vi "Field Data Manager.vi"(6 "Owning Write":bool, 8 "Increment Sequence":bool, 9 "Operation":T4(ring), 10 "Field Value In":T1, 11 "Field ID":T5) -> (0 "Equal":bool, 2 "Field Value Out":T1)   [LabVIEW 2017]
doc: "Implements the data access operations for the variable table. It supports write, read, assign, and setting flags."
uses:
  <vilib>/Rock Robotics/Network Tables/Field ID.ctl
  <vilib>/Rock Robotics/Network Tables/Field Data.ctl
  <vilib>/Rock Robotics/Network Tables/Field Type.ctl
  <vilib>/Rock Robotics/Network Tables/Sequence.ctl
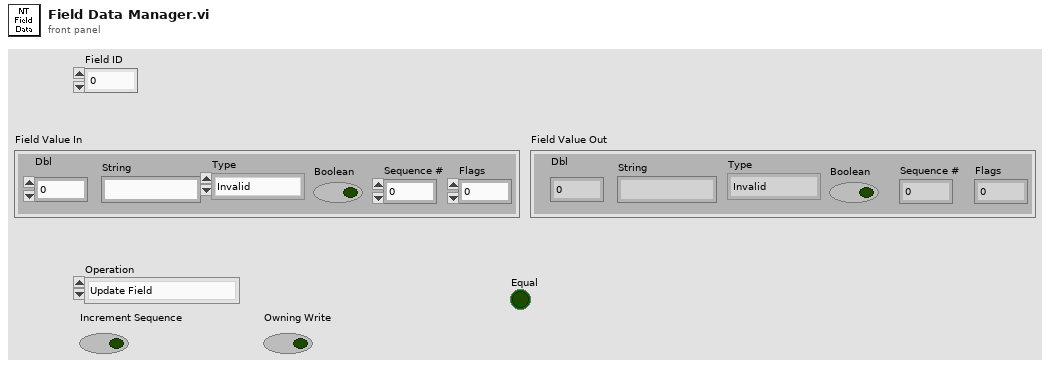
[diagram p1: front panel]
types:
  T1 = typedef "Field Data.ctl" = cluster{"Dbl":dbl, "String":string, "Type":T2, "Boolean":bool, "Sequence #":T3, "Flags":u8}
  T2 = typedef "Field Type.ctl" = enum8{"Invalid", "Bool", "Numeric", "String", "Raw", "Boolean Array", "Numeric Array", "String Array", "RPC"}
  T3 = typedef "Sequence.ctl" = u16
  T4 = enum16{"Update Field", "Read Field", "Assign Field", "Remove All", "Set Persistence", "Clear Persistence"}
  T5 = typedef "Field ID.ctl" = i32
  T6 = cluster{"Dbl":bool, "String":bool, "Type":bool, "Boolean":bool, "Sequence #":bool, "Flags":bool}
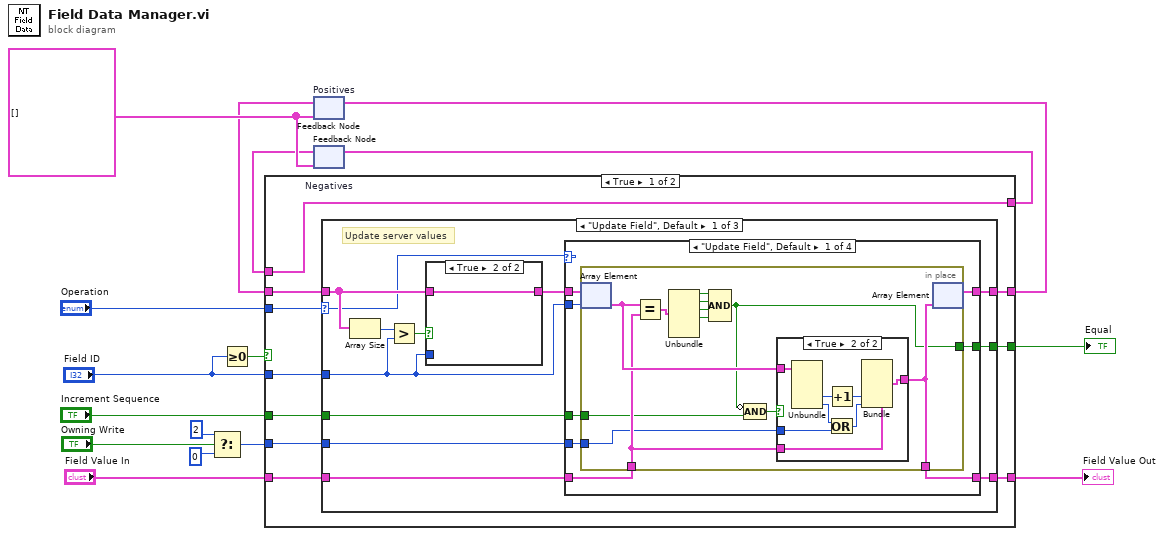
[diagram p0: block diagram]
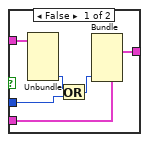
[diagram p2: hidden frame]
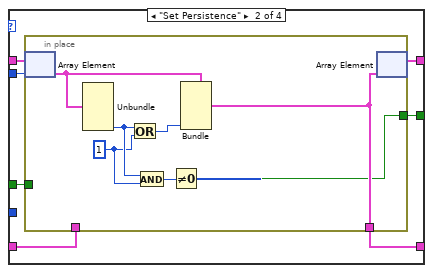
[diagram p3: hidden frame]
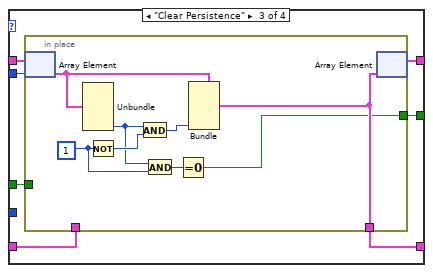
[diagram p4: hidden frame]
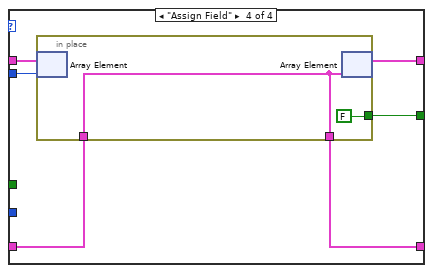
[diagram p5: hidden frame]
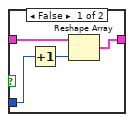
[diagram p6: hidden frame]
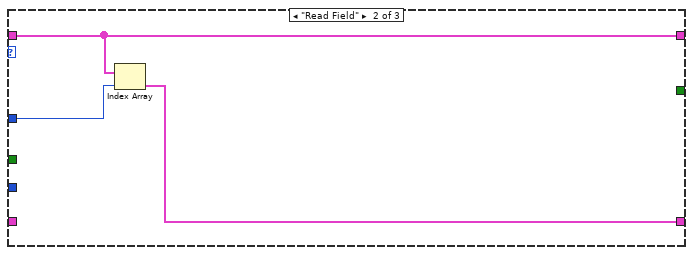
[diagram p7: hidden frame]
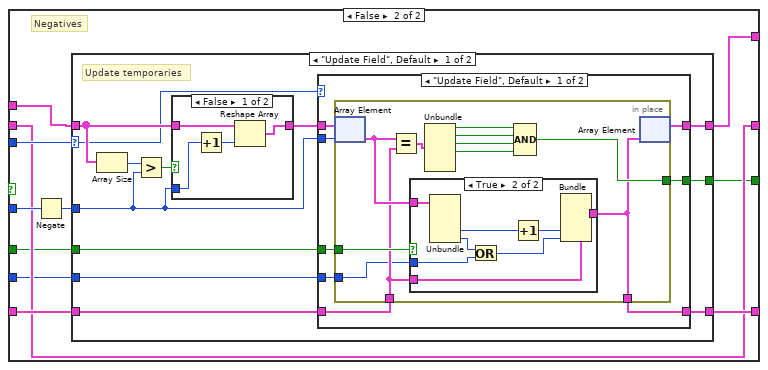
[diagram p9: hidden frame]
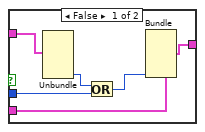
[diagram p10: hidden frame]
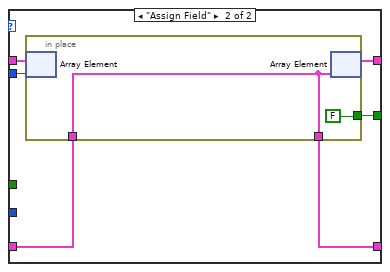
[diagram p11: hidden frame]
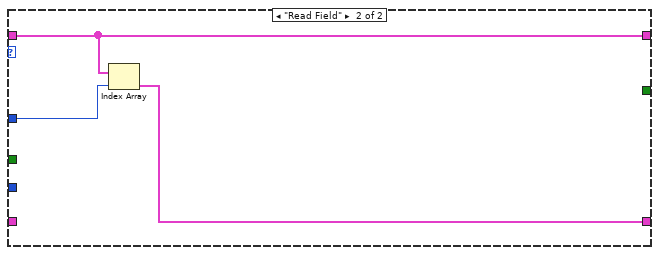
[diagram p13: hidden frame]
diagram:
  w12 = T1[] []
  n1 = Select(t=u8 2, s="Owning Write", f=u8 0) -> (s? t:f=w1:u8)
  n2 = Greater Or Equal To 0?(x="Field ID") -> (x >= 0?=w5:bool)
  n3 = feedback #1 "Positives"(w12) -> (w9:T1[])
  n4 = feedback #2 "Negatives"(w12) -> (w7:T1[])
  n5 = case shown="True" w5 {
    tunnel: "Operation" -> [w26 w129]
    tunnel: "Field Value In" -> [w25 w128]
    tunnel: w9 -> [w24 w123]
    tunnel: [w23 w127] -> w14
    tunnel: [w22 w123] -> w8
    tunnel: "Field ID" -> [w21 w126]
    tunnel: [w20 w124] -> w6
    tunnel: w7 -> [w20 w125]
    tunnel: [w19 w121] -> w11
    tunnel: "Increment Sequence" -> [w18 w120]
    tunnel: w1 -> [w17 w119]
    frame True {
      n6 = case shown="\"Update Field\", Default" w26 {
        selector: w26 -> [w29 _ _]
        tunnel: w25 -> [w36 _ w118]
        tunnel: w24 -> [w34 w115 _]
        tunnel: w21 -> [w31 w117 _]
        tunnel: [w37 w116 w118] -> w23
        tunnel: [w35 w115 _] -> w22
        tunnel: [w30 _ _] -> w19
        tunnel: w18 -> [w28 _ _]
        tunnel: w17 -> [w27 _ _]
        frame "Update Field", Default {
          # "Update server values"
          n7 = Array Size(array=w34) -> (size(s)=w38:i32)
          n8 = Greater?(x=w38, y=w31) -> (0:w32:bool)
          n9 = case shown="True" w32 {
            tunnel: [w112 w114] -> w33
            tunnel: w34 -> [w113 w114]
            tunnel: w31 -> [w111 _]
            frame False {
              n10 = Increment(x=w111) -> (x+1=w110:T5)
              n11 = Reshape Array(w113, w110) -> (w112:T1[])
            }
            frame True {
            }
          }
          n12 = case shown="\"Update Field\", Default" w29 {
            tunnel: [w46 w79 w93 w107] -> w37
            tunnel: w36 -> [w45 w78 w92 w106]
            tunnel: [w44 w77 w91 w105] -> w35
            tunnel: w33 -> [w43 w76 w90 w104]
            tunnel: w31 -> [w42 w75 w89 w103]
            tunnel: [w41 w73 w88 w102] -> w30
            tunnel: w28 -> [w40 w74 w87 _]
            tunnel: w27 -> [w39 _ _ _]
            frame "Update Field", Default {
              n13 = in-place {
                in-place-border: w45 -> [w52]
                in-place-border: [w51] -> w46
                in-place-border: [w48] -> w41
                in-place-border: w40 -> [w50]
                in-place-border: w39 -> [w47]
                n14 = in-place-array #3(w43, w42) -> (w53:T1)
                n15 = Equal?(x=w53, y=w52) -> (x = y?=w58:T6)
                n16 = Unbundle(w58) -> ("Dbl"=w54:bool, "String"=w55:bool, "Type"=w56:bool, "Boolean"=w57:bool)  [unwired: 2 out]
                n17 = Compound Arithmetic op=AND(w54, w55, w56, w57) -> (w48:bool)
                n18 = Compound Arithmetic op=AND(invert w48, w50) -> (w49:bool)
                n19 = case shown="True" w49 {
                  tunnel: w53 -> [w63 w72]
                  tunnel: w52 -> [w64 w71]
                  tunnel: [w62 w70] -> w51
                  tunnel: w47 -> [w61 w67]
                  frame False {
                    n20 = Unbundle(w63) -> ("Flags"=w60:u8)  [unwired: 5 out]
                    n21 = Or(x=w60, y=w61) -> (x .or. y?=w59:u8)
                    n22 = Bundle(cluster=w64, "Flags"=w59) -> (w62:T1)  [unwired: 5 in]
                  }
                  frame True {
                    n23 = Unbundle(w72) -> ("Sequence #"=w69:T3, "Flags"=w66:u8)  [unwired: 4 out]
                    n24 = Increment(x=w69) -> (x+1=w68:T3)
                    n25 = Or(x=w66, y=w67) -> (x .or. y?=w65:u8)
                    n26 = Bundle(cluster=w71, "Sequence #"=w68, "Flags"=w65) -> (w70:T1)  [unwired: 4 in]
                  }
                }
                n27 = in-place-array #3(w51) -> (w44:T1[])  [unwired: 1 out]
              }
            }
            frame "Set Persistence" {
              n28 = in-place {
                in-place-border: w78 -> [_]
                in-place-border: [w86] -> w79
                in-place-border: w74 -> [_]
                in-place-border: [w80] -> w73
                w82 = u8 1 ("Flags")
                n29 = in-place-array #4(w76, w75) -> (w85:T1)
                n30 = Unbundle(w85) -> ("Flags"=w83:u8)  [unwired: 5 out]
                n31 = Or(x=w83, y=w82) -> (x .or. y?=w84:u8)
                n32 = And(x=w83, y=w82) -> (x .and. y?=w81:u8)
                n33 = Not Equal To 0?(x=w81) -> (x != 0?=w80:bool)
                n34 = Bundle(cluster=w85, "Flags"=w84) -> (w86:T1)  [unwired: 5 in]
                n35 = in-place-array #4(w86) -> (w77:T1[])  [unwired: 1 out]
              }
            }
            frame "Clear Persistence" {
              n36 = in-place {
                in-place-border: w92 -> [_]
                in-place-border: [w101] -> w93
                in-place-border: [w94] -> w88
                in-place-border: w87 -> [_]
                w96 = u8 1 ("Flags")
                n37 = in-place-array #5(w90, w89) -> (w100:T1)
                n38 = Unbundle(w100) -> ("Flags"=w97:u8)  [unwired: 5 out]
                n39 = Not(x=w96) -> (.not. x?=w98:u8)
                n40 = And(x=w97, y=w98) -> (x .and. y?=w99:u8)
                n41 = And(x=w97, y=w96) -> (x .and. y?=w95:u8)
                n42 = Equal To 0?(x=w95) -> (x = 0?=w94:bool)
                n43 = Bundle(cluster=w100, "Flags"=w99) -> (w101:T1)  [unwired: 5 in]
                n44 = in-place-array #5(w101) -> (w91:T1[])  [unwired: 1 out]
              }
            }
            frame "Assign Field" {
              n45 = in-place {
                in-place-border: w106 -> [w108]
                in-place-border: [w108] -> w107
                in-place-border: [FALSE] -> w102
                n46 = in-place-array #6(w104, w103) -> ()  [unwired: 1 out]
                n47 = in-place-array #6(w108) -> (w105:T1[])  [unwired: 1 out]
              }
            }
          }
        }
        frame "Read Field" {
          n48 = Index Array(array=w115, index=w117) -> (element=w116:T1)
        }
        frame "Remove All" {
        }
      }
    }
    frame False {
      # "Negatives"
      n49 = Negate(x=w126) -> (-x=w122:T5)
      n50 = case shown="\"Update Field\", Default" w129 {
        selector: w129 -> [w133 _]
        tunnel: w128 -> [w138 _]
        tunnel: w125 -> [w140 w188]
        tunnel: w122 -> [w134 w190]
        tunnel: [w132 w189] -> w127
        tunnel: [w136 w188] -> w124
        tunnel: [w137 _] -> w121
        tunnel: w120 -> [w131 _]
        tunnel: w119 -> [w130 _]
        frame "Update Field", Default {
          # "Update temporaries"
          n51 = Array Size(array=w140) -> (size(s)=w141:i32)
          n52 = Greater?(x=w141, y=w134) -> (0:w139:bool)
          n53 = case shown="False" w139 {
            tunnel: [w185 w187] -> w135
            tunnel: w140 -> [w186 w187]
            tunnel: w134 -> [w184 _]
            frame False {
              n54 = Increment(x=w184) -> (x+1=w183:T5)
              n55 = Reshape Array(w186, w183) -> (w185:T1[])
            }
            frame True {
            }
          }
          n56 = case shown="\"Update Field\", Default" w133 {
            tunnel: [w149 w180] -> w132
            tunnel: w138 -> [w148 w179]
            tunnel: [w147 w178] -> w136
            tunnel: w135 -> [w146 w177]
            tunnel: w134 -> [w145 w176]
            tunnel: [w144 w175] -> w137
            tunnel: w131 -> [w143 _]
            tunnel: w130 -> [w142 _]
            frame "Update Field", Default {
              n57 = in-place {
                in-place-border: w148 -> [w152]
                in-place-border: [w151] -> w149
                in-place-border: [w155] -> w144
                in-place-border: w143 -> [w154]
                in-place-border: w142 -> [w150]
                n58 = in-place-array #7(w146, w145) -> (w153:T1)
                n59 = Equal?(x=w153, y=w152) -> (x = y?=w160:T6)
                n60 = case shown="True" w154 {
                  tunnel: w153 -> [w166 w174]
                  tunnel: w152 -> [w165 w173]
                  tunnel: [w164 w172] -> w151
                  tunnel: w150 -> [w161 w169]
                  frame False {
                    n61 = Unbundle(w166) -> ("Flags"=w163:u8)  [unwired: 5 out]
                    n62 = Or(x=w163, y=w161) -> (x .or. y?=w162:u8)
                    n63 = Bundle(cluster=w165, "Flags"=w162) -> (w164:T1)  [unwired: 5 in]
                  }
                  frame True {
                    n64 = Unbundle(w174) -> ("Sequence #"=w171:T3, "Flags"=w168:u8)  [unwired: 4 out]
                    n65 = Or(x=w168, y=w169) -> (x .or. y?=w167:u8)
                    n66 = Increment(x=w171) -> (x+1=w170:T3)
                    n67 = Bundle(cluster=w173, "Sequence #"=w170, "Flags"=w167) -> (w172:T1)  [unwired: 4 in]
                  }
                }
                n68 = Unbundle(w160) -> ("Dbl"=w156:bool, "String"=w157:bool, "Type"=w158:bool, "Boolean"=w159:bool)  [unwired: 2 out]
                n69 = Compound Arithmetic op=AND(w156, w157, w158, w159) -> (w155:bool)
                n70 = in-place-array #7(w151) -> (w147:T1[])  [unwired: 1 out]
              }
            }
            frame "Assign Field" {
              n71 = in-place {
                in-place-border: w179 -> [w181]
                in-place-border: [w181] -> w180
                in-place-border: [FALSE] -> w175
                n72 = in-place-array #8(w177, w176) -> ()  [unwired: 1 out]
                n73 = in-place-array #8(w181) -> (w178:T1[])  [unwired: 1 out]
              }
            }
          }
        }
        frame "Read Field" {
          n74 = Index Array(array=w188, index=w190) -> (element=w189:T1)
        }
      }
    }
  }
  "Field Value Out" <- w14
  "Equal" <- w11
  n75 = feedback-in #1(w8) -> ()
  n76 = feedback-in #2(w6) -> ()
